vi "Convert Module Name to Type.vi"(8 "error in (no error)":errorcluster, 11 "Module in":refnum<class "Module.lvclass">) -> (0 "error out":errorcluster, 3 "Module out":refnum<class "Module.lvclass">)   [LabVIEW 2015, in "Module.lvclass"]
uses:
  Module.lvclass
  Module.lvclass/Module.ctl
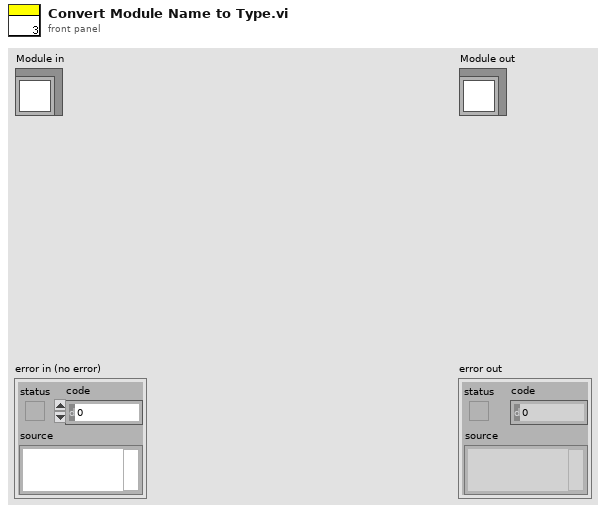
[diagram p1: front panel]
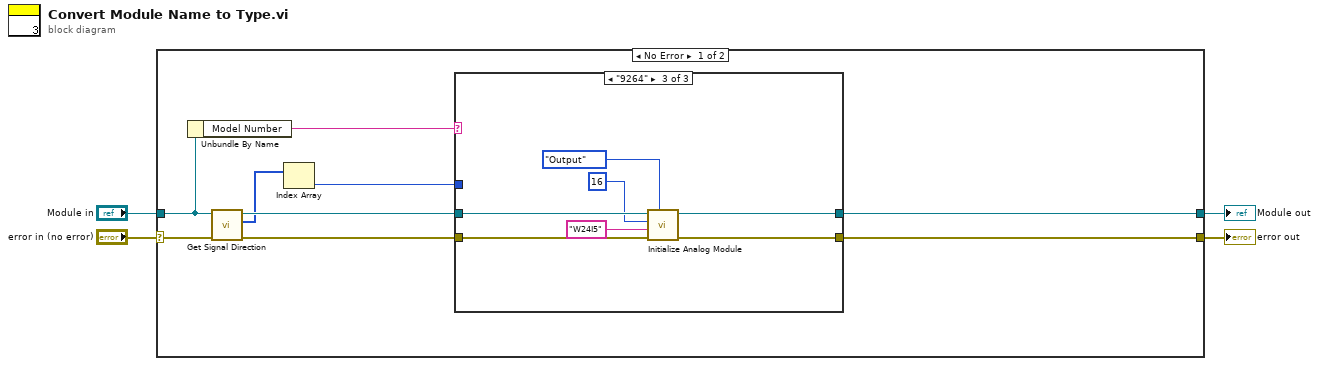
[diagram p0: block diagram]
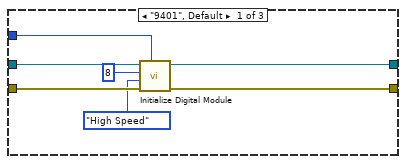
[diagram p2: hidden frame]
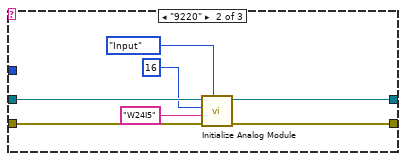
[diagram p3: hidden frame]
diagram:
  n1 = case shown="No Error" "error in (no error)" {
    selector: "error in (no error)" -> [w10 w36]
    tunnel: [w12 w36] -> w3
    tunnel: [w13 w35] -> w1
    tunnel: "Module in" -> [w8 w35]
    frame No Error {
      n2 = Unbundle By Name(w8) -> ("Model Number"=w11:string)
      n3 = call "Get Signal Direction.vi"("error in (no error)"=w10, "Module in"=w8) -> ("error out"=w9:errorcluster, "Direction"=w6:enum16{"Input", "Output"}[], "Module out"=w7:refnum<class "Module.lvclass">)  [unwired: 7 in]
      n4 = Index Array(array=w6) -> (element=w5:enum16{"Input", "Output"})  [unwired: 1 in]
      n5 = case shown="\"9264\"" w11 {
        tunnel: w7 -> [w20 w27 w34]
        tunnel: [w19 w26 w33] -> w13
        tunnel: w9 -> [w18 w25 w32]
        tunnel: [w17 w24 w31] -> w12
        tunnel: w5 -> [w14 _ _]
        frame "9401", Default {
          n6 = call "Initialize Digital Module.vi"("Direction"=w14, "error in (no error)"=w18, "Speed"=enum16{"High Speed", "Low Speed"}."High Speed", "Channels"=u8 8, "Module in"=w20) -> ("error out"=w17:errorcluster, "Module out"=w19:refnum<class "Module.lvclass">)  [unwired: 5 in]
        }
        frame "9220" {
          n7 = call "Initialize Analog Module.vi"("Direction"=enum16{"Input", "Output"}."Input", "error in (no error)"=w25, "FXP Type"="W24I5", "Channels"=u8 16, "Module in"=w27) -> ("error out"=w24:errorcluster, "Module out"=w26:refnum<class "Module.lvclass">)  [unwired: 5 in]
        }
        frame "9264" {
          n8 = call "Initialize Analog Module.vi"("Direction"=enum16{"Input", "Output"}."Output", "error in (no error)"=w32, "FXP Type"="W24I5", "Channels"=u8 16, "Module in"=w34) -> ("error out"=w31:errorcluster, "Module out"=w33:refnum<class "Module.lvclass">)  [unwired: 5 in]
        }
      }
    }
    frame Error {
    }
  }
  "error out" <- w3
  "Module out" <- w1
